vi "AMySubViHelper.vi"(8 "Fehler (Eingang, kein Fehler)":errorcluster, 11 "VI (Eingang)":refnum<vi>) -> (0 "Fehler (Ausgang)":errorcluster, 1 "WhereIGetMyInformation":string, 2 "WhoIAm":string)   [LabVIEW 2013]
uses:
  ApplicationInititialisationClass/ApplicationInititialisation.lvclass
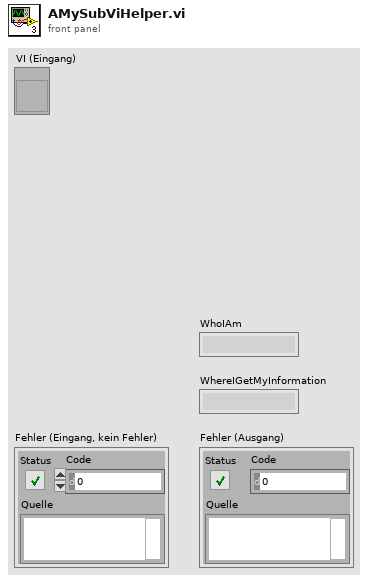
[diagram p1: front panel]
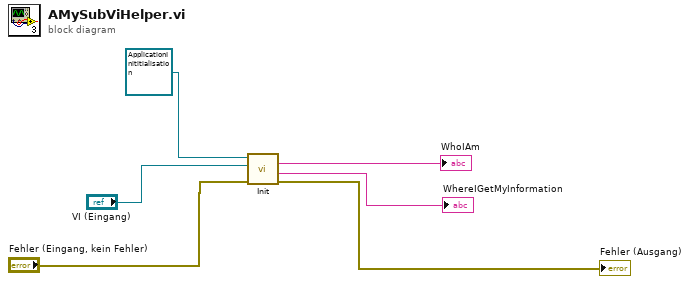
[diagram p0: block diagram]
diagram:
  n1 = call-dynamic "Init.vi"("error in (no error)"="Fehler (Eingang, kein Fehler)", "Main Vi Reference 2"="VI (Eingang)", "ApplicationInititialisation Eingang"=refnum<class "ApplicationInititialisation.lvclass"> refnum ("ApplicationInititialisation.lvclass")) -> ("error out"=→"Fehler (Ausgang)":errorcluster, "WhereIGetMyInformation"=→"WhereIGetMyInformation":string, "WhoIAm"=→"WhoIAm":string)  [unwired: 5 in, 1 out]
